vi "TEST CalcSweepPoints.vi"() -> ()   [LabVIEW 2017]
panel:
  out "Waveform Graph":dbl[][](graph)
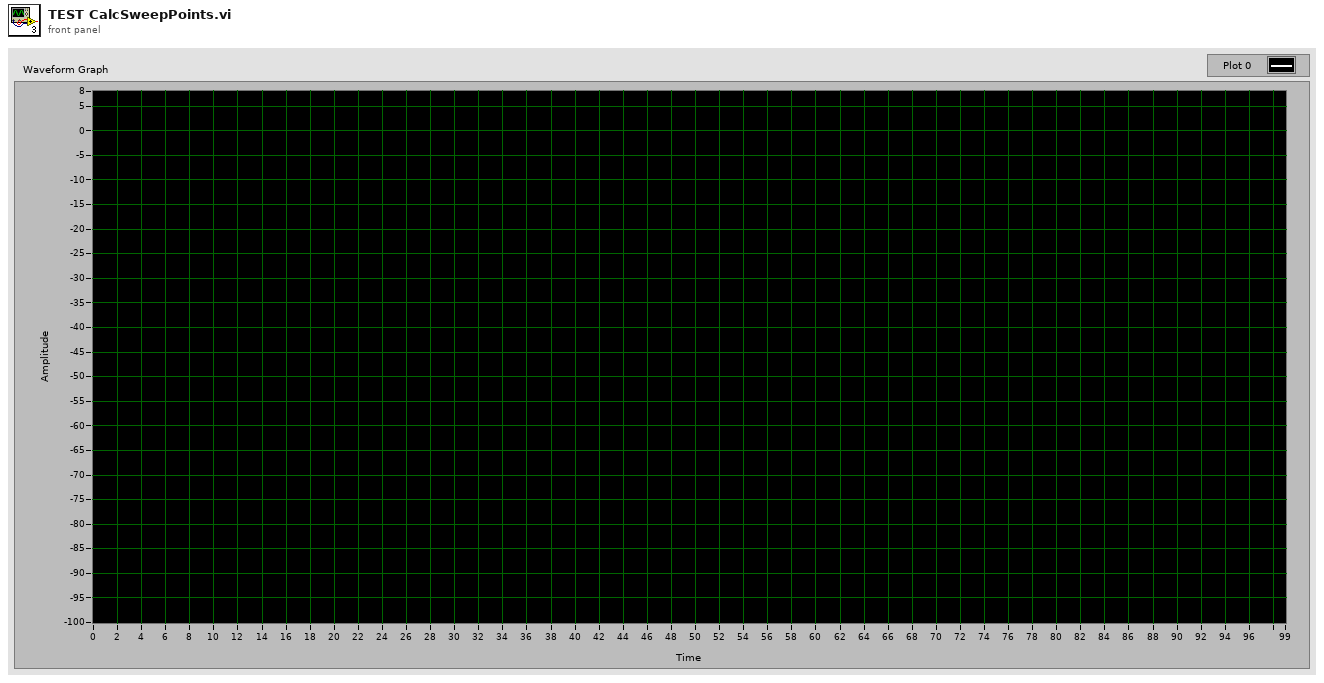
[diagram p1: front panel]
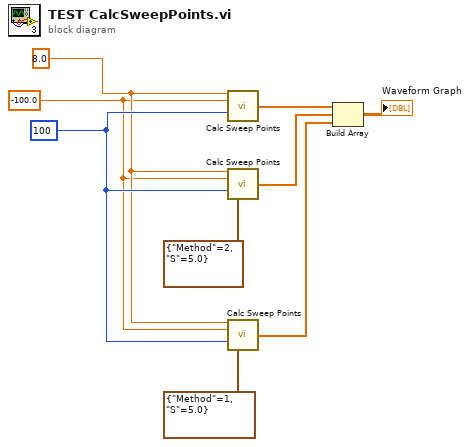
[diagram p0: block diagram]
diagram:
  w4 = 100 ("Points(0 as default)\"")
  w2 = -100.0 ("Start")
  w3 = 8.0 ("Start")
  n1 = call "Calc Sweep Points.vi"("Start"=w3, "Stop(Use \"Span\" if it's not NaN)"=w2, "Points(0 as default)\""=w4) -> ("SweepPoints"=w9:dbl[])  [unwired: 12 in]
  n2 = call "Calc Sweep Points.vi"("Start"=w3, "Stop(Use \"Span\" if it's not NaN)"=w2, "Points(0 as default)\""=w4, "Setting"=cluster{"Method":u16, "S":dbl} {"Method"=2, "S"=5.0}) -> ("SweepPoints"=w6:dbl[])  [unwired: 11 in]
  n3 = call "Calc Sweep Points.vi"("Start"=w3, "Stop(Use \"Span\" if it's not NaN)"=w2, "Points(0 as default)\""=w4, "Setting"=cluster{"Method":u16, "S":dbl} {"Method"=1, "S"=5.0}) -> ("SweepPoints"=w1:dbl[])  [unwired: 11 in]
  n4 = Build Array(w9, w6, w1) -> (→"Waveform Graph":dbl[][])
